vi "Tell Init Child.vi"(4 "Unified Actor Alias":string, 7 "Actor in":refnum<class "Actor.lvclass">, 9 "Msg":T1 {"Teller"."Absolute Time" format="%<%x %.3X>T"}) -> (0 "Error out":errorcluster, 1 "Told":bool, 5 "Actor out":refnum<class "Actor.lvclass">)   [LabVIEW 2020, in "jettl.lvlib"]
uses:
  jettl.lvlib
  Msg/Msg.lvclass
  Actor/Actor.lvclass
  Msg Input/Msg Input.lvclass
  Msg Output/Msg Output.lvclass
  Unified Actor Relation.ctl
  Teller.ctl
  Msg.ctl
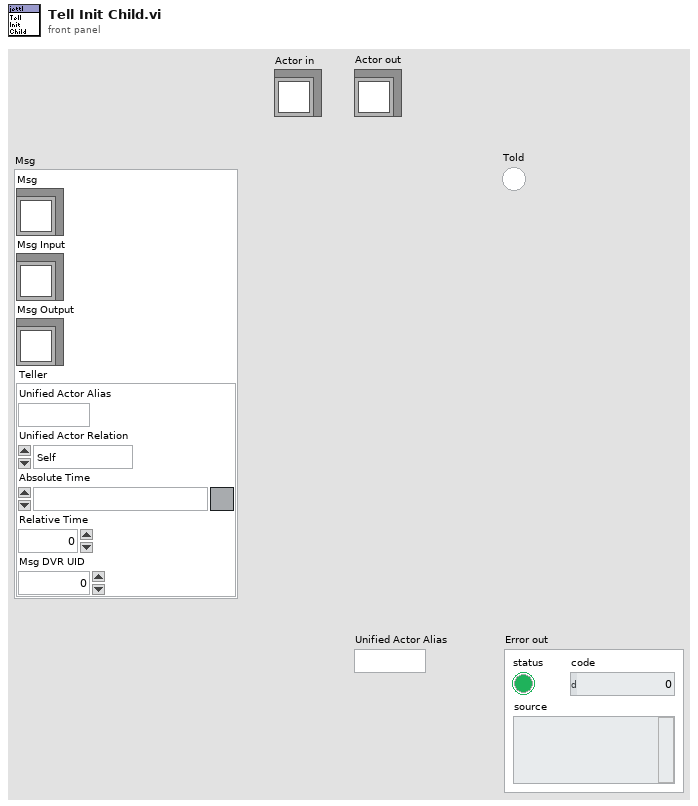
[diagram p1: front panel]
types:
  T1 = typedef "jettl.lvlib/Msg.ctl" = cluster{"Msg":refnum<class "Msg.lvclass">, "Msg Input":refnum<class "Msg Input.lvclass">, "Msg Output":refnum<class "Msg Output.lvclass">, "Teller":T2}
  T2 = typedef "jettl.lvlib/Teller.ctl" = cluster{"Unified Actor Alias":string, "Unified Actor Relation":T3, "Absolute Time":timestamp, "Relative Time":dbl, "Msg DVR UID":i32}
  T3 = typedef "jettl.lvlib/Unified Actor Relation.ctl" = enum16{"Self", "Parent", "Child"}
  T4 = typedef "jettl.lvlib/Unified Actor.ctl" = cluster{"Msgs":T5, "Leaf":bool, "Edge Actors":refnum<class "Actor.lvclass">[], "Core Actors":refnum<class "Actor.lvclass">[], "Root":bool, "Alias":string, "DVR UID":i32, "Transport":refnum<user-event>, "Address":refnum<event-registration>, "This VI":refnum<vi>}
  T5 = typedef "jettl.lvlib/Msgs.ctl" = cluster{"Inbound":T6, "Outbound":T6, "Implemented":T6, "Tell Init":T6, "Tell Init Self":T6, "Tell Init Parent":T6, "Tell Init Child":T6, "Tell Forward":T6, "Tell Forward Self":T6, "Tell Forward Parent":T6, "Tell Forward Child":T6}
  T6 = typedef "jettl.lvlib/Msg Set.ctl" = set{refnum<class "Msg.lvclass">}
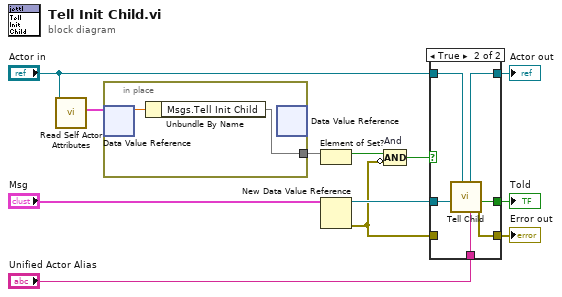
[diagram p0: block diagram]
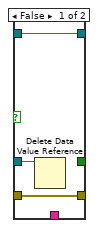
[diagram p2: hidden frame]
diagram:
  n1 = call-dynamic "Read Self Actor Attributes.vi"("Actor in"="Actor in") -> ("Self Actor Attributes"=w7:T4)  [unwired: 10 in]
  n2 = in-place {
    in-place-border: [w13] -> w6
    n3 = in-place-dvr #1(w7) -> (w14:dbl)  [unwired: 1 out]
    n4 = Unbundle By Name(w14) -> ("Msgs.Tell Init Child"=w13)
    n5 = in-place-dvr #1() -> ()  [unwired: 1 in, 2 out]
  }
  n6 = Element of Set?(11:w6) -> (3:w3:bool)  [unwired: 1 in]
  n7 = New Data Value Reference(data value="Msg") -> (data value reference=w12:refnum<data-value>, error out=w4:errorcluster)  [unwired: 1 in]
  n8 = Compound Arithmetic op=AND "And"(w3, invert w4) -> (w2:bool)
  n9 = case shown="True" w2 {
    tunnel: w12 -> [w16 w21]
    tunnel: [w17 w19] -> w9
    tunnel: "Actor in" -> [w15 w23]
    tunnel: [w15 w22] -> w11
    tunnel: [_ w20] -> w10
    tunnel: "Unified Actor Alias" -> [_ w18]
    tunnel: w4 -> [w17 _]
    frame False {
      n10 = Delete Data Value Reference(data value reference=w16) -> ()  [unwired: 1 in, 2 out]
    }
    frame True {
      n11 = call "Tell Child.vi"("Unified Actor Alias"=w18, "Actor in"=w23, "Msg DVR"=w21) -> ("Error out"=w19:errorcluster, "Told"=w20:bool, "Actor out"=w22:refnum<class "Actor.lvclass">)  [unwired: 6 in]
    }
  }
  "Error out" <- w9
  "Actor out" <- w11
  "Told" <- w10
